vi "mfd_global_v2.0.vi"() -> ()   [LabVIEW 2023]
panel:
  out "MFD_Gps 2":picture
  out "MFD_HW":T1={"Tittle"="   HW-STAT", "Sensors"=["3D ACC", "3D GYRO", "3D MAG", "ABS PRES", "DIFF PRESS", "GPS", "OPTICAL FLOW", "ANGULAR CONT", "ATT STAB", "YAW POSITION", "Z ALT CONTR", "XY POS CONTR", "MOTORs", "RC RECEIVER", "AHRS", "TERRAIN", "LOGGING", "BATTERY", "SATCOM", "ARM CHECK"], "P"={"3D ACC"=FALSE, "3D GYRO"=FALSE, "3D MAG"=FALSE, "ABS PRESS"=FALSE, "DIFF PRESS"=FALSE, "GPS"=FALSE, "OPTICAL FLOW"=FALSE, "ANGULAR RATE"=FALSE, "ATT STAB"=FALSE, "YAW POSS"=FALSE, "Z ALT CONTR"=FALSE, "3D ACC 12"=FALSE, "Motors"=FALSE, "RC RECEIVER"=FALSE, "AHRS"=FALSE, "TERRAIN"=FALSE, "BATTERY"=FALSE, "LOGGING"=FALSE, "SATCOM"=FALSE, "ARM CHECK"=FALSE}, "E"={"3D ACC"=FALSE, "3D GYRO"=FALSE, "3D MAG"=FALSE, "ABS PRESS"=FALSE, "DIFF PRESS"=FALSE, "GPS"=FALSE, "OPTICAL FLOW"=FALSE, "ANGULAR RATE"=FALSE, "ATT STAB"=FALSE, "YAW POSS"=FALSE, "Z ALT CONTR"=FALSE, "3D ACC 12"=FALSE, "Motors"=FALSE, "RC RECEIVER"=FALSE, "AHRS"=FALSE, "TERRAIN"=FALSE, "BATTERY"=FALSE, "LOGGING"=FALSE, "SATCOM"=FALSE, "ARM CHECK"=FALSE}, "H"={"3D ACC"=FALSE, "3D GYRO"=FALSE, "3D MAG"=FALSE, "ABS PRESS"=FALSE, "DIFF PRESS"=FALSE, "GPS"=FALSE, "OPTICAL FLOW"=FALSE, "ANGULAR RATE"=FALSE, "ATT STAB"=FALSE, "YAW POSS"=FALSE, "Z ALT CONTR"=FALSE, "3D ACC 12"=FALSE, "Motors"=FALSE, "RC RECEIVER"=FALSE, "AHRS"=FALSE, "TERRAIN"=FALSE, "BATTERY"=FALSE, "LOGGING"=FALSE, "SATCOM"=FALSE, "ARM CHECK"=FALSE}, "usage=s"=0, "usage"="MLP time", "free mem"="Free mem (b)", "heap top"="Heap top (b)", "usage="=0.0, "free_mem=s"=0, "free_mem= "=0.0} {"free_mem=s" scale=0.0..1000.0; "usage=s" scale=0.0..1000.0}
  out "MFD_StatusText":cluster{"Tittle":string, "Status Text":string[]}={"Tittle"=" STATUS TEXT", "Status Text"=[""]}
  out "MFD_Gps":T2={"Tittle"="    GPS", "GPS_FIX="="NO GPS", "LAT"="LAT", "LAT="="-", "LON"="LON", "LON="="-", "Tittle_Pos"="   POSITION", "title__"=["GPS FIX", "SATs", "HDOP", "VDOP", "ALT", "GS", "CoG"], "SATs=s"=12, "SATs="=0, "HDOP="="-", "\nVDOP="="-", "ALT="="-", "GS="="-", "Cogs="="-"} {"SATs=s" scale=0.0..20.0}
  out "MFD_RadioBattery":T3={"Tittle_Power"=" POWER", "Tittle_Radio"=" RADIO", "RSSI"="RSSI = 0", "CH"="CHs = 0", "VCC"="VCC = 0 V", "VSERVO"="Servo = 0 V", "BRICK"=FALSE, "SERVO"=FALSE, "USB"=FALSE, "Peripheral OC"=FALSE, "Peripheral  HI OC"=FALSE, "Status Changed"=FALSE, "Tittle_Battery"=" BATTERY", "Batt_v"="V = 0 V", "Bat_I"="I = 0 A", "Bat_Temp"="T = 0", "1"=1000, "2"=1000, "3"=1000, "4"=1000, "5"=1000, "6"=1000, "7"=1000, "8"=1000, "9"=1000, "10"=1000, "11"=1000, "12"=1000, "13"=1000, "14"=1000, "15"=1000, "16"=1000, "Battery%"=0, "faults"={"DD"=FALSE, "S"=FALSE, "CF"=FALSE, "OC"=FALSE, "OT"=FALSE, "UT"=FALSE, "IV"=FALSE, "IF"=FALSE}} {"Battery%" scale=0.0..100.0; "16" scale=1000.0..2000.0; "15" scale=1000.0..2000.0; "14" scale=1000.0..2000.0; "13" scale=1000.0..2000.0; "12" scale=1000.0..2000.0; "11" scale=1000.0..2000.0; "10" scale=1000.0..2000.0; "9" scale=1000.0..2000.0; "8" scale=1000.0..2000.0; "7" scale=1000.0..2000.0; "6" scale=1000.0..2000.0; "5" scale=1000.0..2000.0; "4" scale=1000.0..2000.0; "3" scale=1000.0..2000.0; "2" scale=1000.0..2000.0; "1" scale=1000.0..2000.0}
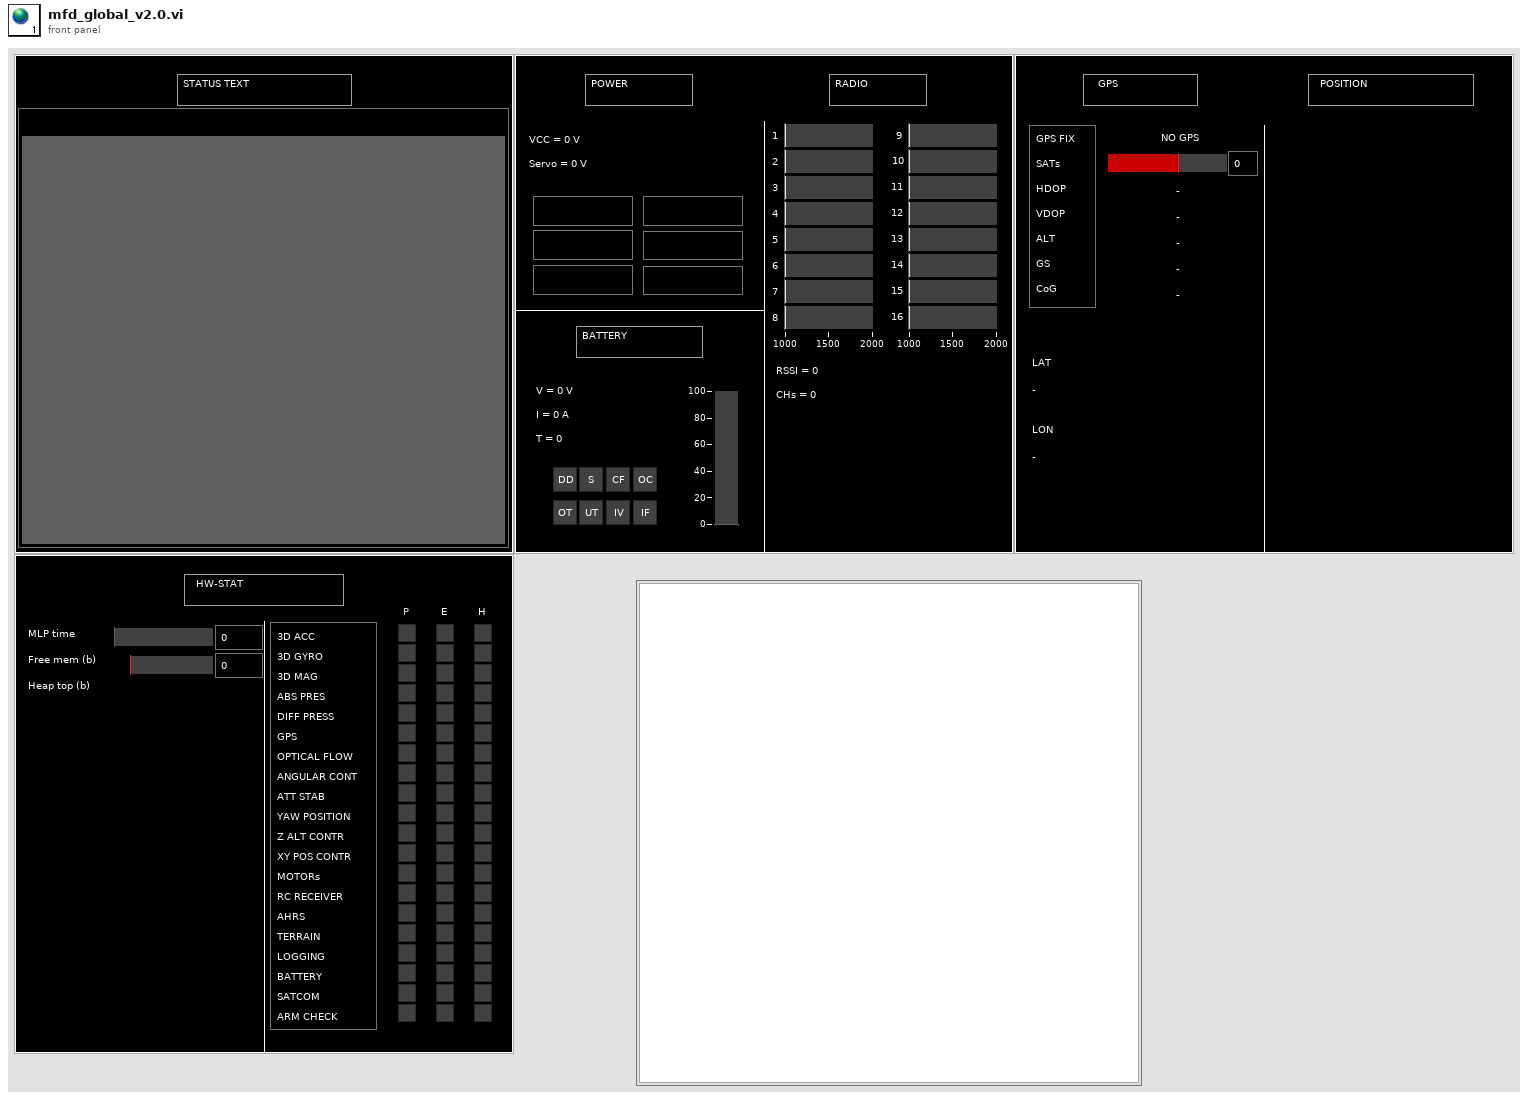
[diagram p1: front panel]
types:
  T1 = cluster{"Tittle":string, "Sensors":string[], "P":cluster{"3D ACC":bool, "3D GYRO":bool, "3D MAG":bool, "ABS PRESS":bool, "DIFF PRESS":bool, "GPS":bool, "OPTICAL FLOW":bool, "ANGULAR RATE":bool, "ATT STAB":bool, "YAW POSS":bool, "Z ALT CONTR":bool, "3D ACC 12":bool, "Motors":bool, "RC RECEIVER":bool, "AHRS":bool, "TERRAIN":bool, "BATTERY":bool, "LOGGING":bool, "SATCOM":bool, "ARM CHECK":bool}, "E":cluster{"3D ACC":bool, "3D GYRO":bool, "3D MAG":bool, "ABS PRESS":bool, "DIFF PRESS":bool, "GPS":bool, "OPTICAL FLOW":bool, "ANGULAR RATE":bool, "ATT STAB":bool, "YAW POSS":bool, "Z ALT CONTR":bool, "3D ACC 12":bool, "Motors":bool, "RC RECEIVER":bool, "AHRS":bool, "TERRAIN":bool, "BATTERY":bool, "LOGGING":bool, "SATCOM":bool, "ARM CHECK":bool}, "H":cluster{"3D ACC":bool, "3D GYRO":bool, "3D MAG":bool, "ABS PRESS":bool, "DIFF PRESS":bool, "GPS":bool, "OPTICAL FLOW":bool, "ANGULAR RATE":bool, "ATT STAB":bool, "YAW POSS":bool, "Z ALT CONTR":bool, "3D ACC 12":bool, "Motors":bool, "RC RECEIVER":bool, "AHRS":bool, "TERRAIN":bool, "BATTERY":bool, "LOGGING":bool, "SATCOM":bool, "ARM CHECK":bool}, "usage=s":u16, "usage":string, "free mem":string, "heap top":string, "usage=":sgl, "free_mem=s":u16, "free_mem= ":sgl}
  T2 = cluster{"Tittle":string, "GPS_FIX=":string, "LAT":string, "LAT=":string, "LON":string, "LON=":string, "Tittle_Pos":string, "title__":string[], "SATs=s":u8, "SATs=":u8, "HDOP=":string, "\nVDOP=":string, "ALT=":string, "GS=":string, "Cogs=":string}
  T3 = cluster{"Tittle_Power":string, "Tittle_Radio":string, "RSSI":string, "CH":string, "VCC":string, "VSERVO":string, "BRICK":bool, "SERVO":bool, "USB":bool, "Peripheral OC":bool, "Peripheral  HI OC":bool, "Status Changed":bool, "Tittle_Battery":string, "Batt_v":string, "Bat_I":string, "Bat_Temp":string, "1":u16, "2":u16, "3":u16, "4":u16, "5":u16, "6":u16, "7":u16, "8":u16, "9":u16, "10":u16, "11":u16, "12":u16, "13":u16, "14":u16, "15":u16, "16":u16, "Battery%":i8, "faults":cluster{"DD":bool, "S":bool, "CF":bool, "OC":bool, "OT":bool, "UT":bool, "IV":bool, "IF":bool}}
diagram:
